vi "DigitalOut_write.vi"(8 "error in (no error)":errorcluster, 9 "Value":bool, 11 "DigitalOut in":refnum<class "DigitalOut.lvclass">) -> (0 "error out":errorcluster, 3 "DigitalOut out":refnum<class "DigitalOut.lvclass">)   [LabVIEW 2011, in "mbed_LVLibrary.lvlib" / "DigitalOut.lvclass"]
uses:
  DigitalOut.lvclass
  DigitalOut.lvclass/DigitalOut.ctl
  Transport Mechanisms/mbed/mbed.lvclass
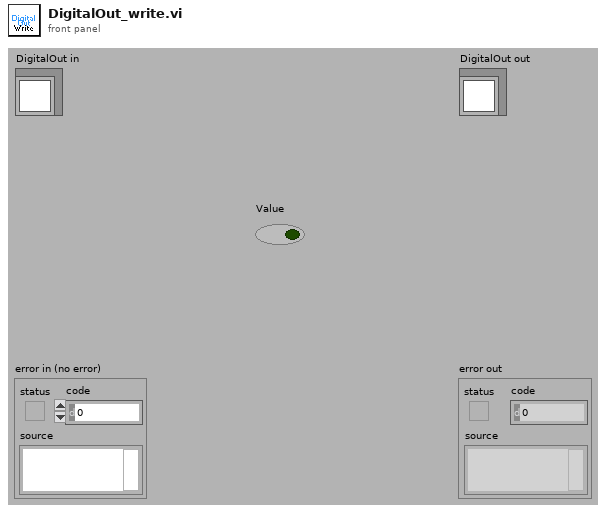
[diagram p1: front panel]
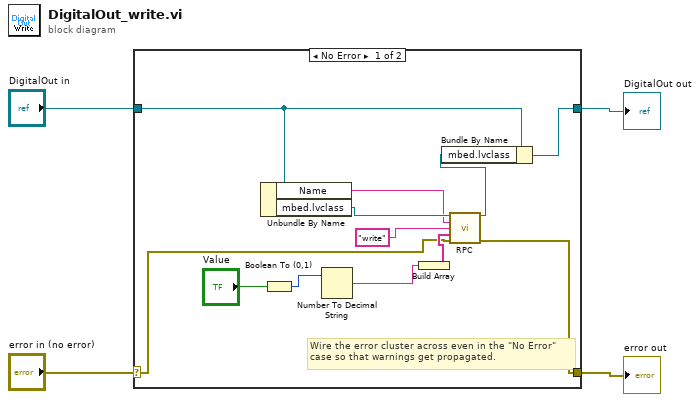
[diagram p0: block diagram]
diagram:
  n1 = case shown="No Error" "error in (no error)" {
    selector: "error in (no error)" -> [w6 w18]
    tunnel: [w5 w18] -> w3
    tunnel: [w8 w17] -> w1
    tunnel: "DigitalOut in" -> [w9 w17]
    frame No Error {
      # "Wire the error cluster across even in the \"No Error\"\ncase so that warnings get propagated."
      n2 = Unbundle By Name(w9) -> ("Name"=w14:string, "mbed.lvclass"=w16:refnum<class "mbed.lvclass">)
      n3 = Boolean To (0,1)(Boolean="Value") -> (0, 1=w12:i16)
      n4 = Number To Decimal String(number=w12) -> (decimal integer string=w11:string)  [unwired: 1 in]
      n5 = Build Array(w11) -> (w10:string[])
      n6 = call-dynamic "RPC.vi"("mbed in"=w16, "Name"=w14, "method"="write", "Args"=w10, "error in (no error)"=w6) -> ("mbed out"=w7:refnum<class "mbed.lvclass">, "error out"=w5:errorcluster)  [unwired: 8 in, 1 out]
      n7 = Bundle By Name(cluster=w9, "mbed.lvclass"=w7) -> (w8:refnum<class "DigitalOut.lvclass">)
    }
    frame Error {
    }
  }
  "error out" <- w3
  "DigitalOut out" <- w1
